vi "AerotechOpenSynchronization.vi"(9 "error in (no error)":errorcluster) -> (2 "Synchro":T1, 6 "error out":errorcluster)   [LabVIEW 2009]
uses:
  Controls/AerotechSynchro.ctl
  Controls/AerotechCommand.ctl
  Controls/AerotechState.ctl
  Controls/AerotechTarget.ctl
  Controls/AerotechScope.ctl
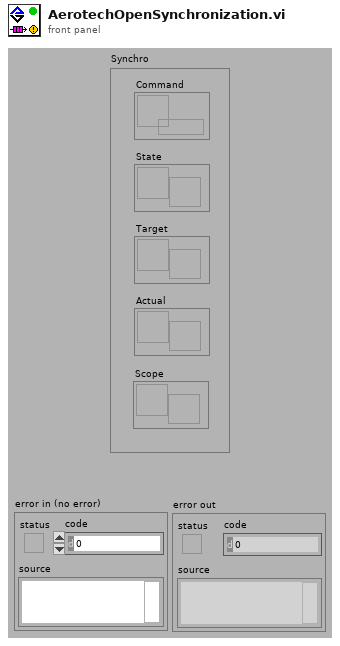
[diagram p1: front panel]
types:
  T1 = typedef "AerotechSynchro.ctl" = cluster{"Command":refnum<queue>, "State":refnum<notifier>, "Target":refnum<notifier>, "Actual":refnum<notifier>, "Scope":refnum<notifier>}
  T2 = typedef "AerotechScope.ctl" = cluster{"First element":i32, "Buffer":i32[]}
  T3 = typedef "AerotechTarget.ctl" = cluster{"Time":timestamp, "Position":dbl, "Velocity":dbl}
  T4 = typedef "AerotechState.ctl" = enum16{"INITING", "IDLING", "SLEWING", "TRACKING", "MOVING", "HOMING", "STOPPING", "RECORDING"}
  T5 = typedef "AerotechCommand.ctl" = enum16{"TRACK", "POSITION", "STOP", "HOME", "QUIT", "RECORD"}
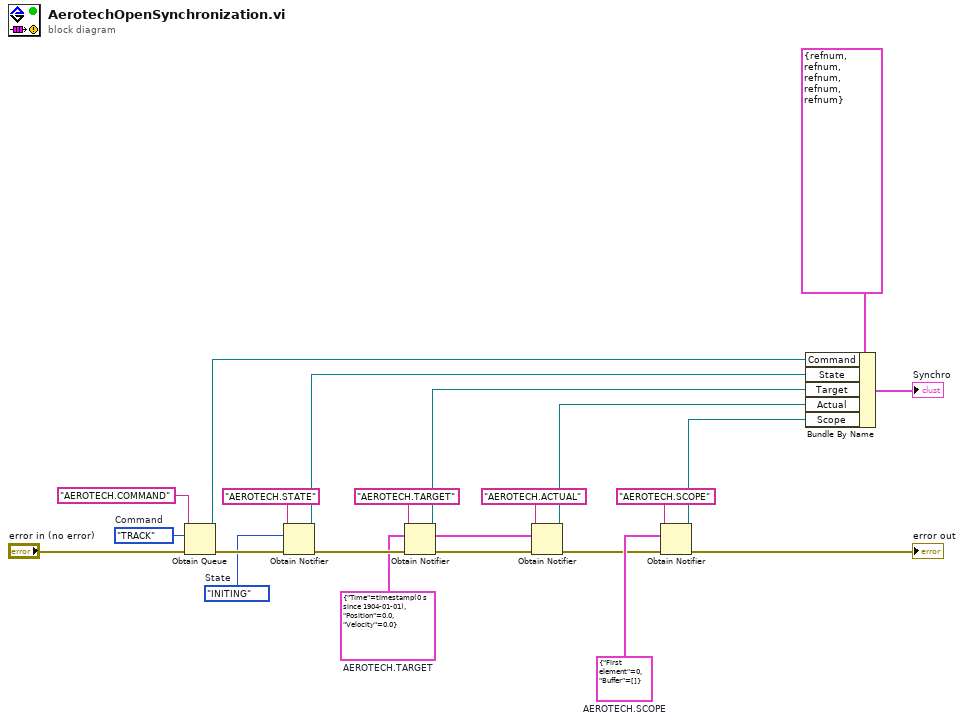
[diagram p0: block diagram]
diagram:
  w4 = T2 {"First element"=0, "Buffer"=[]}  # AEROTECH.SCOPE
  w7 = T3 {"Time"=timestamp(0 s since 1904-01-01), "Position"=0.0, "Velocity"=0.0}  # AEROTECH.TARGET
  w16 = AerotechState."INITING"  # State
  w19 = AerotechCommand."TRACK"  # Command
  n1 = Obtain Queue(name (unnamed)="AEROTECH.COMMAND", element data type=w19, error in (no error)="error in (no error)") -> (queue out=w11:refnum<queue>, error out=w18:errorcluster)  [unwired: 2 in, 1 out]
  n2 = Obtain Notifier(name (unnamed)="AEROTECH.STATE", notification data type=w16, error in (no error)=w18) -> (notifier out=w10:refnum<notifier>, error out=w15:errorcluster)  [unwired: 1 in, 1 out]
  n3 = Obtain Notifier(name (unnamed)="AEROTECH.TARGET", notification data type=w7, error in (no error)=w15) -> (notifier out=w9:refnum<notifier>, error out=w3:errorcluster)  [unwired: 1 in, 1 out]
  n4 = Obtain Notifier(name (unnamed)="AEROTECH.ACTUAL", notification data type=w7) -> (notifier out=w6:refnum<notifier>)  [unwired: 2 in, 2 out]
  n5 = Obtain Notifier(name (unnamed)="AEROTECH.SCOPE", notification data type=w4, error in (no error)=w3) -> (notifier out=w1:refnum<notifier>, error out=→"error out":errorcluster)  [unwired: 1 in, 1 out]
  n6 = Bundle By Name(cluster=T1 {"Command"=refnum, "State"=refnum, "Target"=refnum, "Actual"=refnum, "Scope"=refnum} ("Synchro"), "Command"=w11, "State"=w10, "Target"=w9, "Actual"=w6, "Scope"=w1) -> (→"Synchro":T1)
